vi "Initialize Notifier Controller.vi"(8 "error in (no error)":errorcluster, 9 "Paras In 2":variant, 10 "Paras In":variant, 11 "Simple Map Notifier Controller in":refnum<class "Map Notifier Controller.lvclass">) -> (0 "error out":errorcluster, 3 "Simple Map Notifier Controller out":refnum<class "Map Notifier Controller.lvclass">)   [LabVIEW 2024, in "Map Notifier Controller.lvclass"]
uses:
  Map Notifier Controller.lvclass
  Ancestor Class/Actor Assistant/Notifier/Notifier.lvclass
  Map Notifier Controller.lvclass/Map Notifier Controller.ctl
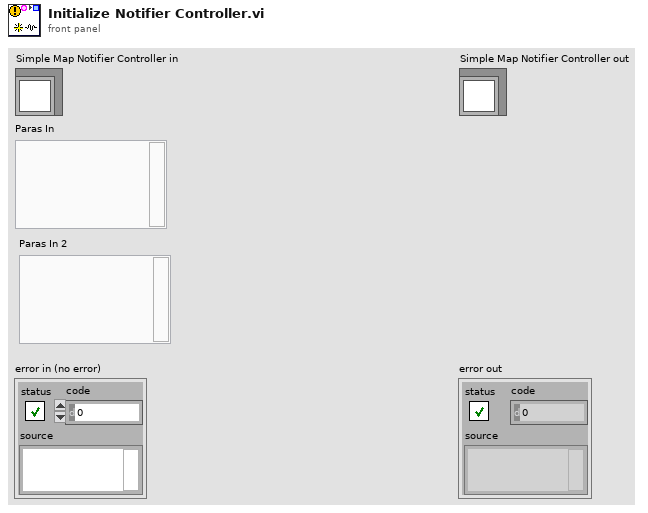
[diagram p1: front panel]
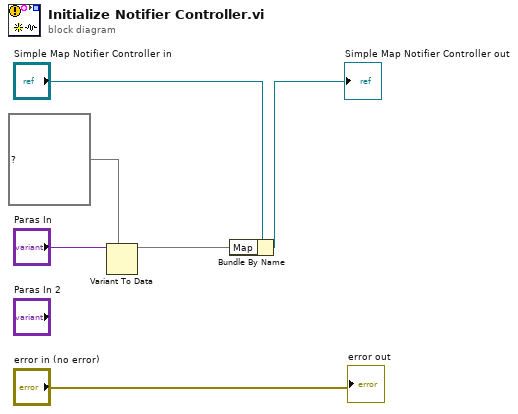
[diagram p0: block diagram]
diagram:
  n1 = Variant To Data(type=map{i64, refnum<class "Notifier.lvclass">} {} ("Map"), Variant="Paras In") -> (data=w1:map{i64, refnum<class "Notifier.lvclass">})  [unwired: 1 in, 1 out]
  n2 = Bundle By Name(cluster="Simple Map Notifier Controller in", "Map"=w1) -> (→"Simple Map Notifier Controller out":refnum<class "Map Notifier Controller.lvclass">)
  "error out" <- "error in (no error)"
